vi "Fault Monitor.vi"() -> ()   [LabVIEW 2023]
doc: "Illustrates how to use the NI Scan Engine Faults VIs to continuously monitor the system for faults, and clear faults."
uses:
  <vilib>/NIScanEngine/faults/Fault.ctl
panel:
  out "Fault List":T1[](array[typedef]) {"level" items=["Minor Fault", "Major Fault", "Unrecoverable Fault"]}
  in  "Stop":bool
  in  "Clear Specific Fault":bool
  in  "Fault Code to Clear":dbl=-66555.0
  in  "Clear All Faults":bool
  # "Overview: Continuously monitor the system for faults and clear a specific fault or all faults.\nRequirements: LabVIEW Real-Time Module and NI-RIO driver\nInstructions:\n1. In Measurement & Automation Explorer, ensure that LabVIEW Real-Time and the NI Scan Engine are installed on your RT target.\n2. From the Project Explorer window, set the IP address of your RT target.\n3. Set the Scan Period (ms) front panel control of either the Timed Loop Synchronization.vi or While Loop Synchronization.vi to the desired loop rate. \n4. Run the VI in which you chose to set the Scan Period (mSec) control. \n5. Use the controls on the front panel to increase the wait amount in the While Loop. When you increase the wait amount beyond the scan period, the loop runs late and LabVIEW generates a fault.\n6. Run Fault Monitor.vi.\n7. Use the controls on the front panel to clear a specific fault code or to clear all faults.\n8. Click the Stop buttons on both VIs."
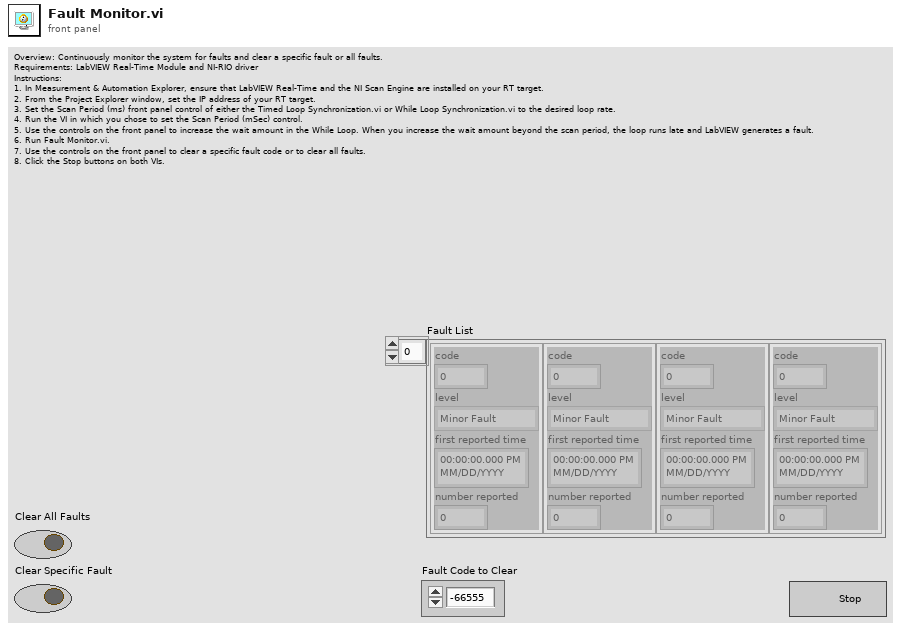
[diagram p1: front panel]
types:
  T1 = typedef "Fault.ctl" = cluster{"code":i32, "level":i32, "first reported time":timestamp, "number reported":u32}
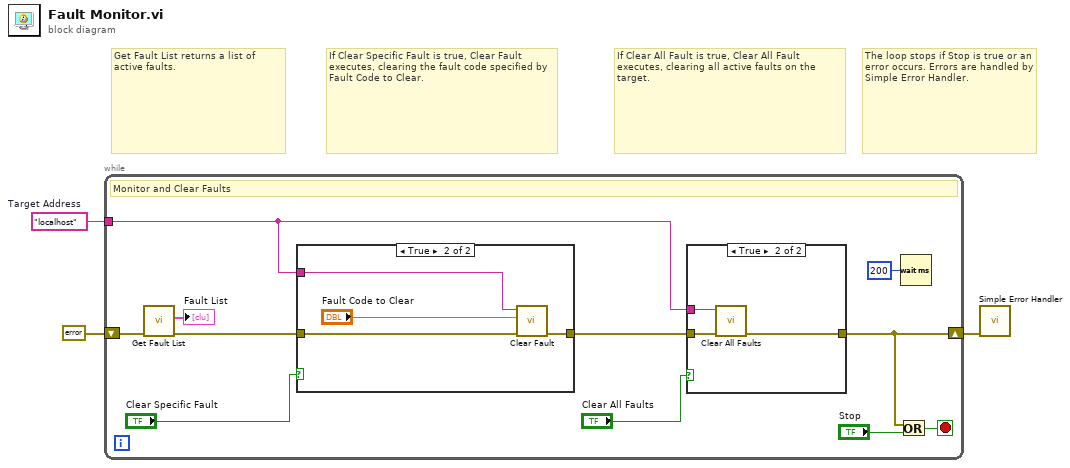
[diagram p0: block diagram]
diagram:
  w3 = "localhost"  # Target Address
  # "The loop stops if Stop is true or an error occurs. Errors are handled by Simple Error Handler."
  # "If Clear All Fault is true, Clear All Fault executes, clearing all active faults on the target."
  # "If Clear Specific Fault is true, Clear Fault executes, clearing the fault code specified by Fault Code to Clear."
  # "Get Fault List returns a list of active faults."
  n1 = while {
    shift-right: [w5] -> w1
    shift-left: errorcluster {"status"=FALSE, "code"=0, "source"=""} ("error in") -> [w14]
    tunnel: w3 -> [w11]
    stop <- w6 stop-if-true
    # "Monitor and Clear Faults"
    n2 = call <vilib>:"Get Fault List.vi"("error in (no error)"=w14) -> ("error out"=w13:errorcluster, "fault list"=→"Fault List":T1[])  [unwired: 9 out]
    n3 = case shown="True" "Clear Specific Fault" {
      tunnel: w13 -> [w19 w23]
      tunnel: [w19 w22] -> w12
      tunnel: w11 -> [_ w21]
      frame False {
      }
      frame True {
        n4 = call <vilib>:"Clear Fault.vi"("error in (no error)"=w23, "fault code"="Fault Code to Clear", "target address (localhost)"=w21) -> ("error out"=w22:errorcluster)  [unwired: 8 out]
      }
    }
    n5 = case shown="True" "Clear All Faults" {
      tunnel: w12 -> [w15 w18]
      tunnel: [w15 w17] -> w5
      tunnel: w11 -> [_ w16]
      frame False {
      }
      frame True {
        n6 = call <vilib>:"Clear All Faults.vi"("error in (no error)"=w18, "target address (localhost)"=w16) -> ("error out"=w17:errorcluster)  [unwired: 9 out]
      }
    }
    n7 = Or(x=w5, y="Stop") -> (x .or. y?=w6:bool)
    n8 = Wait (ms)(milliseconds to wait=u32 200 ("millisecond multiple")) -> ()  [unwired: 1 out]
  }
  n9 = call <vilib>:"Simple Error Handler.vi"("error in (no error)"=w1) -> ()  [unwired: 1 in, 8 out]
